vi "strings.vi"() -> ()   [LabVIEW 2025]
panel:
  in  "name":string
  out "result":string
  in  "age":dbl
  out "date/time string":string
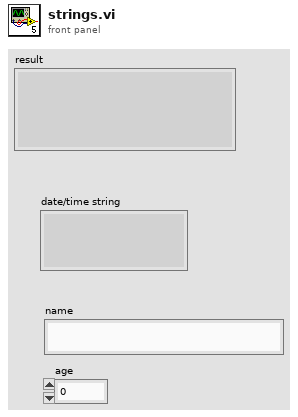
[diagram p1: front panel]
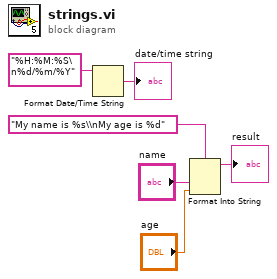
[diagram p0: block diagram]
diagram:
  n1 = Format Date/Time String(time format string (%c)="%H:%M:%S\n%d/%m/%Y") -> (date/time string=→"date/time string":string)  [unwired: 2 in]
  n2 = Format Into String(format string="My name is %s\\nMy age is %d", "name", "age") -> (resulting string=→"result":string)  [unwired: 2 in, 1 out]
